vi "writeToXML.vi"(8 "error in (no error)":errorcluster, 10 "ClassLabel":string, 11 "MccAzElTrack in":refnum<class "MccAzElTrack.lvclass">) -> (0 "error out":errorcluster, 2 "XML out":string, 3 "MccAzElTrack out":refnum<class "MccAzElTrack.lvclass">)   [LabVIEW 2022 SP3, in "TCSDataDefinitions.lvlib" / "TCSMountControlCommand.lvlib" / "CommandsForAzElAxes.lvlib" / "MccAzElTrack.lvclass"]
uses:
  MccAzElTrack.lvclass
  MccAzElTrack.lvclass/MccAzElTrack.ctl
  CommandsForAzElAxes.lvclass
  <userlib>/Common/XML/XMLGenerator/XMLGenerator.lvclass
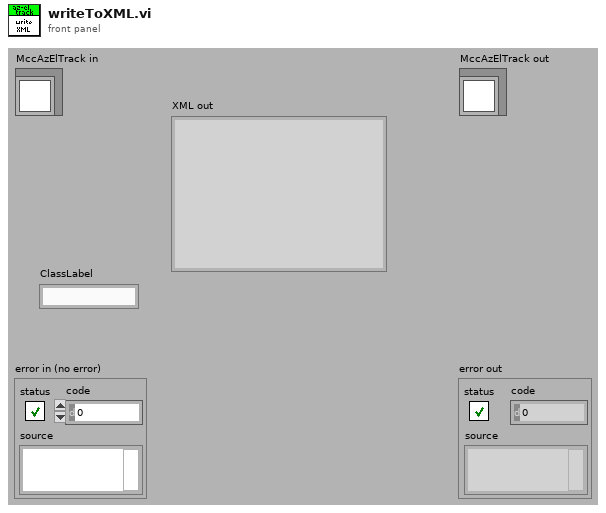
[diagram p1: front panel]
types:
  T1 = typedef "TCSDataDefinitions.lvlib/TCSMountControlCommand.lvlib/MountTrackStates.ctl" = enum16{"On", "Off"}
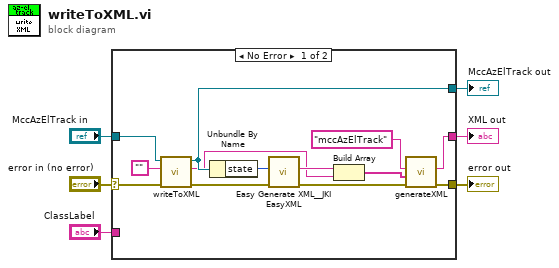
[diagram p0: block diagram]
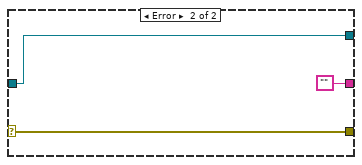
[diagram p2: hidden frame]
diagram:
  n1 = case shown="No Error" "error in (no error)" {
    selector: "error in (no error)" -> [w9 w22]
    tunnel: [w8 w22] -> w5
    tunnel: [w17 w21] -> w3
    tunnel: "MccAzElTrack in" -> [w18 w21]
    tunnel: "ClassLabel" -> [_ _]
    tunnel: [w7 ""] -> w1
    frame No Error {
      n2 = call-parent "writeToXML.vi"("error in (no error)"=w9, "ClassLabel"="", "TCSMCCCommand in"=w18) -> ("error out"=w15:errorcluster, "XMLout"=w13:string, "TCSMCCCommand out"=w17:refnum<class "MccAzElTrack.lvclass">)  [unwired: 6 in]
      n3 = Unbundle By Name(w17) -> ("state"=w16:T1)
      n4 = call <vilib>:"Easy Generate XML__JKI EasyXML.vi"("error in (no error)"=w15, "LabVIEW Data"=w16) -> ("error out"=w10:errorcluster, "XML String"=w14:string)  [unwired: 8 in]
      n5 = Build Array(w14, w13) -> (w12:string[])
      n6 = call <userlib>:"generateXML.vi"("error in"=w10, "childrenXML"=w12, "elementName"="mccAzElTrack" ("Class Label")) -> ("error out"=w8:errorcluster, "XML out"=w7:string)  [unwired: 6 in, 1 out]
    }
    frame Error {
    }
  }
  "error out" <- w5
  "MccAzElTrack out" <- w3
  "XML out" <- w1
